vi "StudentScope - Trigger.vi"(0 "Rate":dbl, 1 "Trigger Slope":bool, 5 "data":dbl[][](array[numeric]), 7 "Level":dbl, 9 "Trigger Channel":u16, 11 "Sec/Div":u32) -> (8 "Array":dbl[][](array[numeric]))   [LabVIEW 2015]
uses:
  <vilib>/measure/mamon.llb/Trigger Detection for 1 Channel (obs).vi
  <vilib>/measure/NI_MAPro.lvlib
panel:
  out "trigger detected?":bool
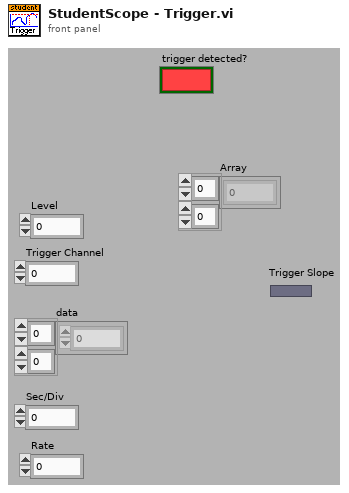
[diagram p1: front panel]
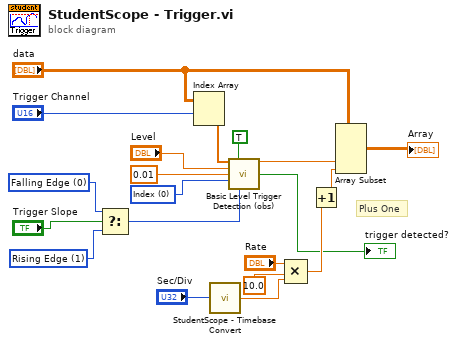
[diagram p0: block diagram]
diagram:
  w6 = u16 0 items=["Falling Edge", "Rising Edge"] ("slope")
  w5 = u16 1 items=["Falling Edge", "Rising Edge"] ("slope")
  w9 = u16 0 items=["Index", "Time"] ("mode")
  # "Plus One"
  n1 = Select(t=w6, s="Trigger Slope", f=w5) -> (s? t:f=w7:u16)
  n2 = Index Array(array="data", index (row)="Trigger Channel") -> (element=w17:dbl[])  [unwired: 1 in]
  n3 = call "StudentScope - Timebase Convert.vi"("Sec/Div"="Sec/Div") -> ("Sec/Div"=w14:dbl)
  n4 = call-poly <vilib>:"Basic Level Trigger Detection (obs).vi"("signal in"=w17, "reset"=TRUE, "level"="Level", "hysteresis"=0.01, "location mode"=w9, "trigger slope"=w7) -> ("trigger location"=w20:dbl, "trigger detected?"=→"trigger detected?":bool)  [unwired: 7 in, 1 out]
  n5 = Compound Arithmetic op=MULTIPLY("Rate", 10.0 ("Rate"), w14) -> (w19:dbl)
  n6 = Increment(x=w19) -> (x+1=w1:dbl)
  n7 = Array Subset(array="data", index (col)=w20, length (col)=w1) -> (→"Array":dbl[][])  [unwired: 2 in]
